vi "Spot Setup.vi"(7 "Spot Frequency (Hz) (20.0)":dbl=20.0 min=20.0 max=30000000.0 step=1.0 format="%.2f", 8 "error in (no error)":errorcluster, 9 "Spot State (F: Off)":bool, 10 "Spot Number (1)":i16=1 min=1 max=7 step=1, 11 "VISA resource name":refnum<visa-resource-name>) -> (0 "error out":errorcluster, 3 "VISA resource name out":refnum<visa-resource-name>)   [LabVIEW 2015, in "Agilent 428X Series.lvlib"]
doc: "This function sets the specified frequency point correction (FREQ1-FREQ7)."
uses:
  Agilent 428X Series.lvlib
panel:
  # "On\nOff"
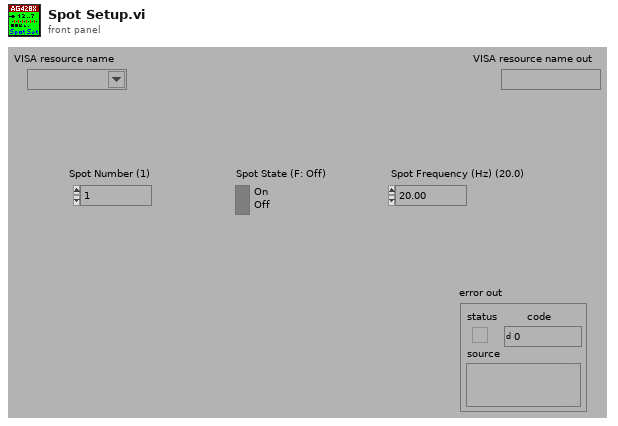
[diagram p1: front panel]
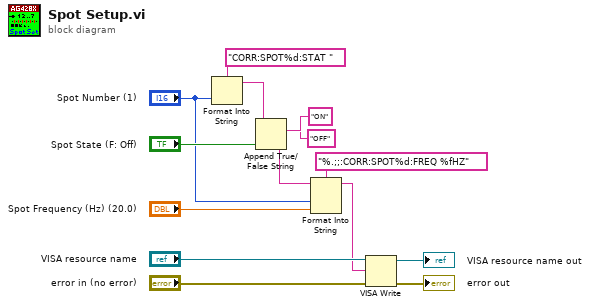
[diagram p0: block diagram]
diagram:
  n1 = Format Into String(format string="CORR:SPOT%d:STAT ", "Spot Number (1)") -> (resulting string=w11:string)  [unwired: 2 in, 1 out]
  n2 = Append True/False String(1:"Spot State (F: Off)", 2:"OFF" ("false string"), 3:"ON" ("true string"), 4:w11) -> (0:w9:string)
  n3 = Format Into String(format string="%.;;:CORR:SPOT%d:FREQ %fHZ", initial string=w9, "Spot Number (1)", "Spot Frequency (Hz) (20.0)") -> (resulting string=w1:string)  [unwired: 1 in, 1 out]
  n4 = VISA Write(VISA resource name="VISA resource name", write buffer=w1, error in (no error)="error in (no error)") -> (VISA resource name out=→"VISA resource name out":refnum<visa-resource-name>, error out=→"error out":errorcluster)  [unwired: 1 out]
